vi "UMB_buildString.vi"(8 "soft e-stop":bool, 9 "Prop":u8(slide)=7 scale=0.0..14.0, 10 "Rudder":u8(knob)=7, 11 "IR Servo":u8(knob)=7 scale=0.0..14.0) -> (3 "string":string)   [LabVIEW 2012]
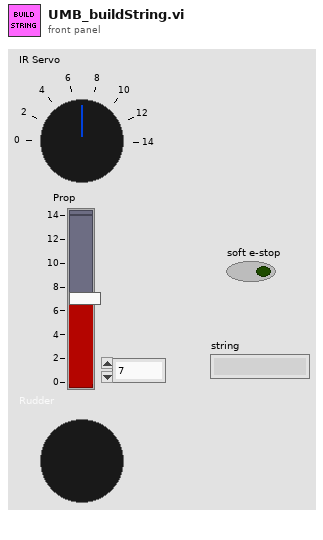
[diagram p1: front panel]
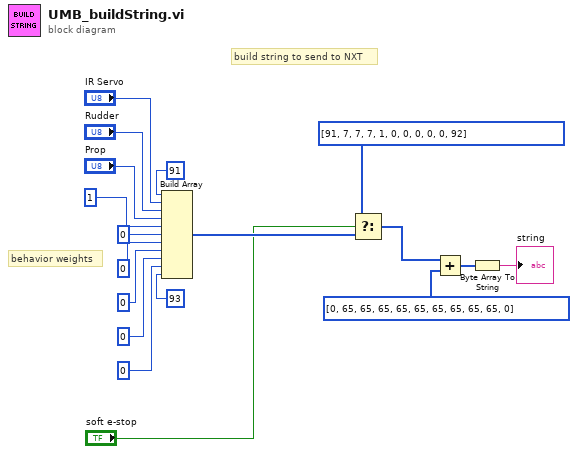
[diagram p0: block diagram]
diagram:
  # "behavior weights"
  # "build string to send to NXT"
  n1 = Build Array(u8 91 ("element"), "IR Servo", "Rudder", "Prop", u8 1 ("# 0"), u8 0 ("# 1"), u8 0 ("# 2"), u8 0 ("# 3"), u8 0 ("# 4"), u8 0 ("# 5"), u8 93 ("element")) -> (w11:u8[])
  n2 = Select(t=u8[] [91, 7, 7, 7, 1, 0, 0, 0, 0, 0, 92], s="soft e-stop", f=w11) -> (s? t:f=w10:u8[])
  n3 = Add(x=w10, y=u8[] [0, 65, 65, 65, 65, 65, 65, 65, 65, 65, 0]) -> (x+y=w9:u8[])
  n4 = Byte Array To String(unsigned byte array=w9) -> (string=→"string":string)
